vi "ClientGetIndividualUDP.vi"(0 "Robot Symbol":string="R") -> (1 "UDP Connection ID":refnum<k16>, 2 "Remote Port #":i32=61540, 3 "error out":errorcluster)   [LabVIEW 2012]
panel:
  out "Valid UDP String?":bool
  out "UDP String":string
  out "Example UDP String":string="$,R,61541,61540,G,61543,61542,B,61545,61544,S,22,1,349\\r"
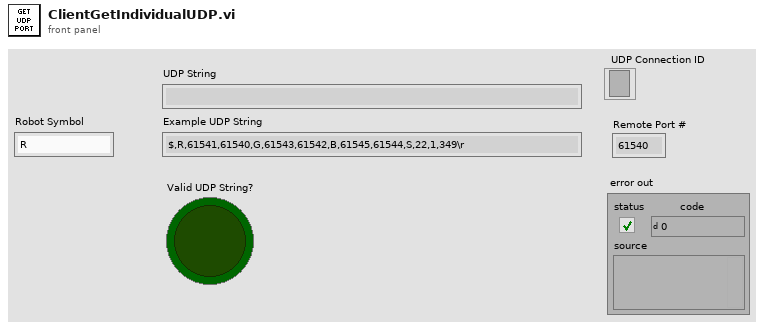
[diagram p1: front panel]
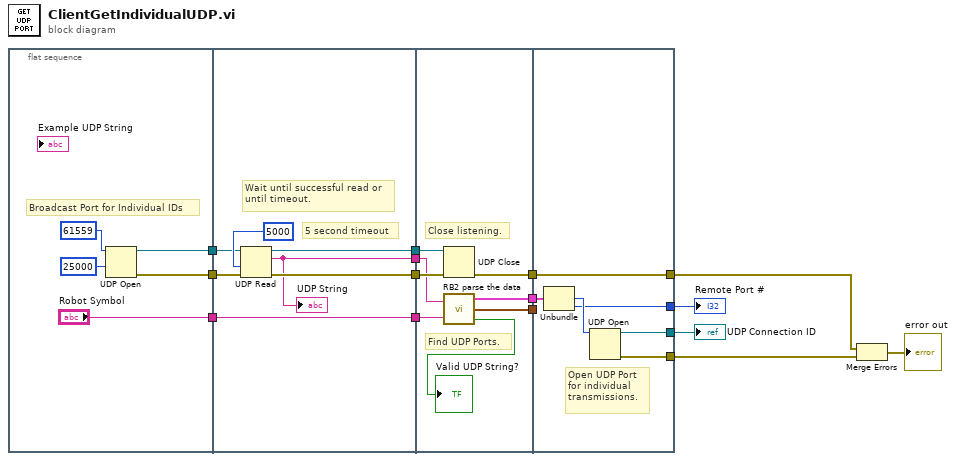
[diagram p0: block diagram]
diagram:
  n1 = flat-sequence {
    tunnel: [w18] -> w14
    tunnel: [w17] -> w13
    tunnel: ["Robot Symbol"] -> w12
    tunnel: w14 -> [w25]
    tunnel: w13 -> [w26]
    tunnel: w12 -> [w22]
    tunnel: [w24] -> w11
    tunnel: [w21] -> w10
    tunnel: [w23] -> w9
    tunnel: [w22] -> w8
    tunnel: w11 -> [w35]
    tunnel: w10 -> [w33]
    tunnel: w9 -> [w34]
    tunnel: w8 -> [w32]
    tunnel: [w31] -> w7
    tunnel: [w30] -> w6
    tunnel: [w29] -> w5
    tunnel: w7 -> [w36]
    tunnel: w6 -> [w41]
    tunnel: w5 -> [_]
    tunnel: [w39] -> w4
    tunnel: [w38] -> w1
    tunnel: [w37] -> w2
    tunnel: [w36] -> w3
    frame #0 {
      # "Broadcast Port for Individual IDs"
      n2 = UDP Open(9:25000 ("timeout ms (25000)"), 11:u16 61559 ("port")) -> (port=w17:refnum<k16>, 0:w18:errorcluster)  [unwired: 3 in, 1 out]
    }
    frame #1 {
      # "5 second timeout"
      # "Wait until successful read or\nuntil timeout."
      n3 = UDP Read(connection ID=w26, timeout ms (25000)=5000, 8:w25) -> (data out=w21:string, error out=w23:errorcluster, 3:w24:refnum<k16>)  [unwired: 1 in, 2 out]
      "UDP String" <- w21
    }
    frame #2 {
      # "Find UDP Ports."
      # "Close listening."
      n4 = UDP Close(connection ID=w35, 8:w34) -> (error out=w31:errorcluster)  [unwired: 1 out]
      n5 = call "RB2 parse the data.vi"("Nav String"=w33, "Jeep"=w32) -> ("Jeep Data"=w30:cluster{"Header":string, i32, i32}, "Time"=w29:cluster{i32, i32, i32}, "Valid?"=→"Valid UDP String?":bool)
    }
    frame #3 {
      # "Open UDP Port\nfor individual\ntransmissions."
      n6 = Unbundle(w41) -> (w40:i32, w39:i32)  [unwired: 1 out]
      n7 = UDP Open(11:w40) -> (port=w38:refnum<k16>, 0:w37:errorcluster)  [unwired: 4 in, 1 out]
    }
  }
  n8 = Merge Errors(w3, w2) -> (→"error out":errorcluster)
  "UDP Connection ID" <- w1
  "Remote Port #" <- w4
